vi "Fgen Arb Sequence.vi"() -> ()   [LabVIEW 2021]
doc: "This example shows how to use Arbitrary Sequence mode. It also shows how you can associate a name with each buffer you are generating."
uses:
  <instrlib>/niFgen/niFgen.llb/niFgen Output Mode.ctl
  <instrlib>/niFgen/niFgen.llb/niFgen_ctl Trigger SW - TrigName Values (Ring).ctl
  <instrlib>/niFgen/niFgen.llb/niFgen Disable Start Trigger.vi
  <instrlib>/niFgen/niFgen.llb/niFgen Configure Software Edge Start Trigger.vi
  <instrlib>/niFgen/niFgen.llb/niFgen Configure Digital Edge Start Trigger.vi
  <instrlib>/niFgen/niFgen.llb/niFgen Create Waveform (I16).vi
panel:
  in  "FGEN Resource Name":refnum<k15>
  in  "Re-Sequence":bool
  in  "Load & Re-Sequence":bool
  out "Resulting Sequence":string[](array[string])
  in  "Digital Filter":bool
  in  "Analog Filter":bool
  in  "DC Offset (V)":dbl(knob) scale=-0.5..0.5 scale format="%#.1f"
  in  "Gain":dbl(knob)=1.0 min=0.0 max=5.0 scale=0.0..5.0 scale format="%#.1f"
  in  "Send Software Trigger":bool
  in  "Sample Clock Source":string(combo)="OnboardClock"
  in  "Clock Mode":u32(ring)=1 items=["Hi Resolution Sampling", "Divide Down Sampling", "Automatic"]
  in  "Trigger Mode":u16(ring)=1 items=["Single", "Continuous", "Stepped", "Burst"]
  in  "Start Trigger Source":string(combo)="PFI0"
  in  "Start Trigger Type":u16(ring) items=["None", "Software Edge", "Digital Edge"]
  in  "Sample Rate":dbl=20000000.0 format="%.2p"
  in  "Sequence":T1(array[cluster])=[{"Waveform Name"=0, "# Loops"=1, "Marker"=-1}, {"Waveform Name"=1, "# Loops"=1, "Marker"=-1}, {"Waveform Name"=2, "# Loops"=3, "Marker"=-1}, {"Waveform Name"=3, "# Loops"=1, "Marker"=-1}] {"Waveform Name" items=["0: Big Ramp", "1: Small Sine", "2: Half Sized Square", "3: DC 0V"]}
  in  "Waveform Information Array":T2(array[cluster])=[{"Name"="Big Ramp", "Waveform"={"Waveform Type"=5, "Amplitude"=1.0, "# of points"=256}}, {"Name"="Small Sine", "Waveform"={"Waveform Type"=0, "Amplitude"=0.5, "# of points"=256}}, {"Name"="Half Sized Square", "Waveform"={"Waveform Type"=3, "Amplitude"=0.5, "# of points"=256}}, {"Name"="DC 0V", "Waveform"={"Waveform Type"=7, "Amplitude"=0.0, "# of points"=256}}] {"Waveform"."Amplitude" min=0.0 max=1.0 format="%.2f"; "Waveform"."Waveform Type" items=["Sine", "Cosine", "Triangle", "Square", "Sawtooth", "Increasing Ramp", "Decreasing Ramp", "DC Value"]}
  in  "Stop Button":bool
  # "Overview: Demonstrates how to configure an NI Arbitrary Waveform Generator to generate an arbitrary waveform with Arbitrary Sequence Mode. This example also demonstrates how to change the sequence without having to reload waveforms to onboard memory\nSoftware Requirements: NI-FGEN\nHardware Requirements: PXI-5411, PCI-5411, AT-5411, PXI-5412, PCI-5412, PXIe-5413, PXI-5421, PCI-5421, PXI-5422, PXIe-5423, PXI-5431, PCI-5431, PXIe-5433, PXI-5441, NI PXIe-5442, NI PXIe-5450, or NI PXIe-5451 \nInstructions:\n1. Select the FGEN Resource Name as configured in the Measurement & Automation Explorer.\n2. Specify the waveforms that will be generated in the Waveform Information Array.\n3. Specify the Sequence that you want to link and loop the waveforms specified in the Waveform Information Array.\n4. Specify the Gain and DC Offset that will be used.\n5. Specify the Sample Rate, Sample Clock Source, and  Clock Mode that will be used.\n6. Select the Start Trigger Type, Trigger Mode, and Start Trigger Source that will be used.\n7. Determine whether to enable the Analog Filter and/or the Digital Filter. \n8. Run the VI.\n9. Click Send Software Trigger to send a trigger if you have selected a relevant Start Trigger Type.\n10. You can change the Gain or DC Offset (V) values on-the-fly. You can also toggle the Analog Filter on-the-fly.\n11. Click Load & Re-Sequence to abort the generation and to load the waveforms from the Waveform Information Array and the Sequence to the device's onboard memory.\n12. Click Re-Sequence to abort the generation and to load the Sequence to the device's onboard memory.\n13. Click Stop to stop the VI."
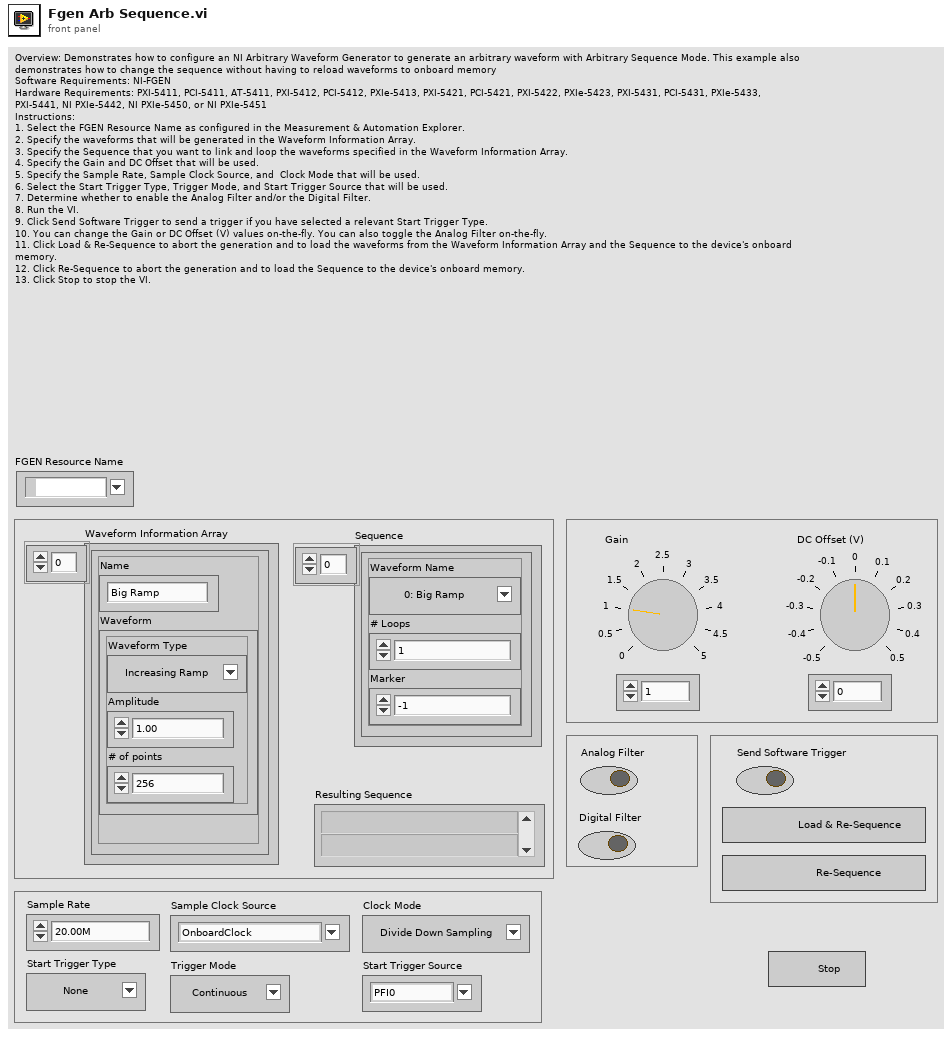
[diagram p1: front panel]
types:
  T1 = cluster{"Waveform Name":u16, "# Loops":i32, "Marker":i32}[]
  T2 = cluster{"Name":string, "Waveform":cluster{"Waveform Type":u16, "Amplitude":dbl, "# of points":u32}}[]
  T3 = typedef "niFgen Output Mode.ctl" = u32
  T4 = cluster{"Waveform Type":u16, "Amplitude":dbl, "# of points":u32}
  T5 = typedef "niFgen_ctl Trigger SW - TrigName Values (Ring).ctl" = i32
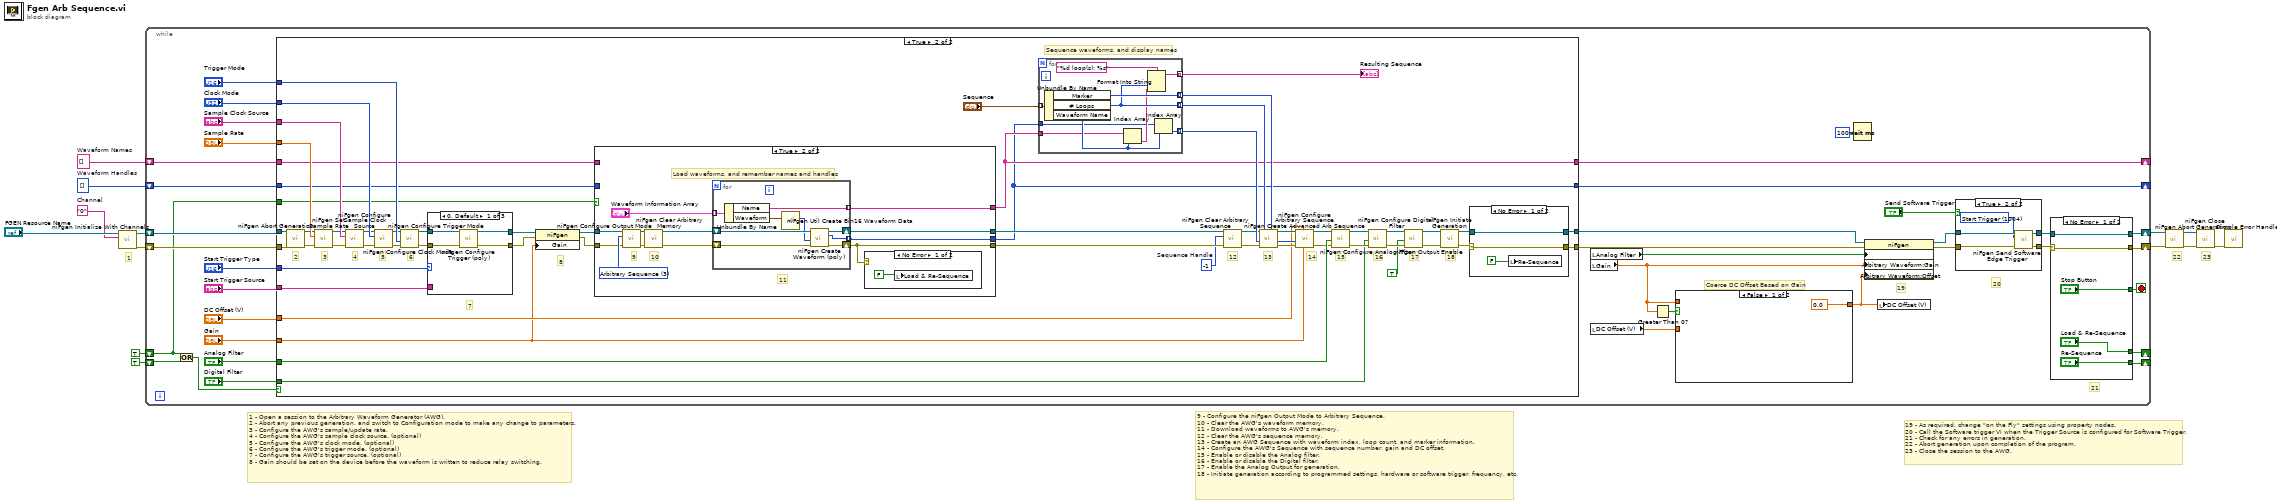
[diagram p0: block diagram]
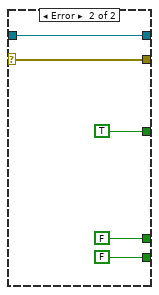
[diagram p2: hidden frame]
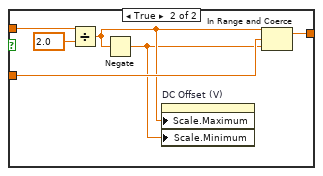
[diagram p3: hidden frame]
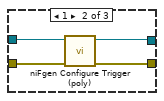
[diagram p9: hidden frame]
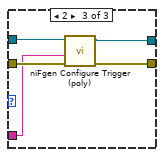
[diagram p10: hidden frame]
diagram:
  w1 = "0"  # Channel
  w9 = i32[] []  # Waveform Handles
  w10 = string[] []  # Waveform Names
  # "1"
  # "23"
  # "22"
  # "19 - As required, change \"on the Fly\" settings using property nodes.\n20 - Call the Software trigger VI when the Trigger Source is configured for Software Trigger.\n21 - Check for any errors in generation.\n22 - Abort generation upon completion of the program. \n23 - Close the session to the AWG."
  # "9 - Configure the niFgen Output Mode to Arbitrary Sequence.\n10 - Clear the AWG's waveform memory.\n11 - Download waveforms to AWG's memory.\n12 - Clear the AWG's sequence memory.\n13 - Create an AWG Sequence with waveform index, loop count, and marker information.\n14 - Configure the AWG's Sequence with sequence number, gain and DC offset.\n15 - Enable or disable the Analog filter.\n16 - Enable or disable the Digital filter.\n17 - Enable the Analog Output for generation.\n18 - Initiate generation according to programmed settings, hardware or software trigger, frequency, etc."
  # "1 - Open a session to the Arbitrary Waveform Generator (AWG).\n2 - Abort any previous generation, and switch to Configuration mode to make any change to parameters.\n3 - Configure the AWG's sample/update rate.\n4 - Configure the AWG's sample clock source. (optional)\n5 - Configure the AWG's clock mode. (optional)\n6 - Configure the AWG's trigger mode. (optional)\n7 - Configure the AWG's trigger source. (optional)\n8 - Gain should be set on the device before the waveform is written to reduce relay switching."
  n1 = call <instrlib>:"niFgen Initialize With Channels.vi"("Channel Name"=w1, "Resource Name"="FGEN Resource Name") -> ("error out"=w2:errorcluster, "Instrument Handle Out"=w3:refnum<k15>)  [unwired: 8 in]
  n2 = while {
    shift-left: TRUE ("Stop Button") -> [w49]
    shift-right: [w27] -> _
    shift-left: TRUE ("Stop Button") -> [w42]
    shift-right: [w28] -> _
    shift-left: w9 -> [w41]
    shift-right: [w38] -> _
    shift-right: [w15] -> w11
    shift-left: w2 -> [w43]
    shift-right: [w39] -> _
    shift-left: w10 -> [w40]
    shift-right: [w16] -> w8
    shift-left: w3 -> [w44]
    stop <- w26 stop-if-true
    # "20"
    # "19"
    # "Coerce DC Offset Based on Gain"
    # "21"
    n3 = Or(x=w42, y=w49) -> (x .or. y?=w50:bool)
    n4 = case shown="True" w50 {
      tunnel: w43 -> [w75 w117]
      tunnel: [w78 w90] -> w37
      tunnel: [w75 w91] -> w36
      tunnel: w44 -> [w78 w116]
      tunnel: "Analog Filter" -> [_ w120]
      tunnel: "Gain" -> [_ w79]
      tunnel: "Sample Rate" -> [_ w106]
      tunnel: "DC Offset (V)" -> [_ w119]
      tunnel: "Start Trigger Type" -> [_ w110]
      tunnel: "Trigger Mode" -> [_ w118]
      tunnel: "Clock Mode" -> [_ w112]
      tunnel: "Digital Filter" -> [_ w115]
      tunnel: "Sample Clock Source" -> [_ w114]
      tunnel: "Start Trigger Source" -> [_ w109]
      tunnel: w42 -> [_ w97]
      tunnel: w41 -> [w76 w95]
      tunnel: w40 -> [w77 w96]
      tunnel: [w77 w94] -> w39
      tunnel: [w76 w85] -> w38
      frame False {
      }
      frame True {
        w87 = -1  # Sequence Handle
        # "8"
        # "Sequence waveforms, and display names"
        # "18"
        # "17"
        # "16"
        # "15"
        # "14"
        # "13"
        # "12"
        # "6"
        # "5"
        # "4"
        # "3"
        # "2"
        # "7"
        n5 = call <instrlib>:"niFgen Abort Generation.vi"("error in (no error)"=w117, "Instrument Handle"=w116) -> ("error out"=w104:errorcluster, "Instrument Handle Out"=w105:refnum<k15>)  [unwired: 8 in]
        n6 = call <instrlib>:"niFgen Set Sample Rate.vi"("error in (no error)"=w104, "Sample Rate (Samp/s)"=w106, "Instrument Handle"=w105) -> ("error out"=w103:errorcluster, "Instrument Handle Out"=w100:refnum<k15>)  [unwired: 7 in]
        n7 = call <instrlib>:"niFgen Configure Sample Clock Source.vi"("error in (no error)"=w103, "Source (Onboard Clock)"=w114, "Instrument Handle"=w100) -> ("error out"=w102:errorcluster, "Instrument Handle Out"=w101:refnum<k15>)  [unwired: 7 in]
        n8 = call <instrlib>:"niFgen Configure Clock Mode.vi"("error in (no error)"=w102, "Clock Mode (default: 1=divide down)"=w112, "Instrument Handle"=w101) -> ("error out"=w111:errorcluster, "Instrument Handle Out"=w113:refnum<k15>)  [unwired: 7 in]
        n9 = call <instrlib>:"niFgen Configure Trigger Mode.vi"("error in (no error)"=w111, "Trigger Mode (default: 1=continuous)"=w118, "Instrument Handle"=w113) -> ("error out"=w130:errorcluster, "Instrument Handle Out"=w81:refnum<k15>)  [unwired: 7 in]
        n10 = case shown="0, Default" w110 {
          tunnel: w130 -> [w170 w174 w179]
          tunnel: [w169 w173 w178] -> w82
          tunnel: w109 -> [_ _ w177]
          tunnel: w81 -> [w168 w172 w176]
          tunnel: [w167 w171 w175] -> w80
          frame 0, Default {
            n11 = call-poly <instrlib>:"niFgen Configure Trigger (poly).vi"("error in (no error)"=w170, "Instrument Handle"=w168) -> ("error out"=w169:errorcluster, "Instrument Handle Out"=w167:refnum<k15>)  [unwired: 8 in]
          }
          frame 1 {
            n12 = call-poly <instrlib>:"niFgen Configure Trigger (poly).vi"("error in (no error)"=w174, "Instrument Handle"=w172) -> ("error out"=w173:errorcluster, "Instrument Handle Out"=w171:refnum<k15>)  [unwired: 8 in]
          }
          frame 2 {
            n13 = call-poly <instrlib>:"niFgen Configure Trigger (poly).vi"("error in (no error)"=w179, "Source"=w177, "Instrument Handle"=w176) -> ("error out"=w178:errorcluster, "Instrument Handle Out"=w175:refnum<k15>)  [unwired: 7 in]
          }
        }
        n14 = property class="niFgen"(reference=w80, error in=w82, "Gain"=w79) -> (reference out=w84:refnum<k15>, error out=w83:errorcluster)
        n15 = case shown="True" w97 {
          tunnel: w84 -> [w144 w153]
          tunnel: w83 -> [w143 w152]
          tunnel: [w143 w149] -> w99
          tunnel: [w144 w147] -> w98
          tunnel: [w141 w151] -> w94
          tunnel: [w142 w148] -> w85
          tunnel: w96 -> [w141 _]
          tunnel: w95 -> [w142 _]
          frame False {
          }
          frame True {
            w154 = T3 3 items=["Standard Function", "Frequency List", "Arbitrary Waveform", "Arbitrary Sequence", "Script"] ("Output Mode")
            # "11"
            # "10"
            # "9"
            # "Load waveforms, and remember names and handles"
            n16 = call <instrlib>:"niFgen Configure Output Mode.vi"("error in (no error)"=w152, "Output Mode (default: 0=Standard Function)"=w154, "Instrument Handle"=w153) -> ("error out"=w155:errorcluster, "Instrument Handle Out"=w156:refnum<k15>)  [unwired: 6 in]
            n17 = call <instrlib>:"niFgen Clear Arbitrary Memory.vi"("error in (no error)"=w155, "Instrument Handle"=w156) -> ("error out"=w146:errorcluster, "Instrument Handle Out"=w145:refnum<k15>)  [unwired: 8 in]
            n18 = for {
              shift-right: [w165] -> w149
              shift-left: w146 -> [w163]
              tunnel: [w158] -> w148 mode=indexing
              shift-right: [w166] -> w147
              shift-left: w145 -> [w164]
              tunnel: [w159] -> w151 mode=indexing
              tunnel: "Waveform Information Array" -> [w160] mode=indexing
              n19 = Unbundle By Name(w160) -> ("Name"=w159:string, "Waveform"=w162:T4)
              n20 = call <instrlib>:"niFgen Util Create Bin16 Waveform Data.vi"("Waveform"=w162) -> ("Waveform Data"=w161:i16[])  [unwired: 10 in]
              n21 = call-poly <instrlib>:"niFgen Create Waveform (poly).vi"("error in (no error)"=w163, "Waveform Data Array"=w161, "Instrument Handle"=w164) -> ("error out"=w165:errorcluster, "Waveform Handle"=w158:i32, "Instrument Handle Out"=w166:refnum<k15>)  [unwired: 6 in]
            }
            n22 = case shown="No Error" w149 {
              frame No Error {
                n23 = local write "Load & Re-Sequence"(FALSE ("Load?")) -> ()
              }
              frame Error {
              }
            }
          }
        }
        n24 = for {
          tunnel: "Sequence" -> [w189] mode=indexing
          tunnel: [w187] -> w132 mode=indexing
          tunnel: [w188] -> w124 mode=indexing
          tunnel: [w185] -> w123 mode=indexing
          tunnel: [w184] -> w88 mode=indexing
          tunnel: w94 -> [w182]
          tunnel: w85 -> [w180]
          n25 = Unbundle By Name(w189) -> ("Marker"=w188:i32, "# Loops"=w185:i32, "Waveform Name"=w183:u16)
          n26 = Index Array(array=w182, index=w183) -> (element=w181:string)
          n27 = Format Into String(format string="%d loop(s): %s", w185, w181) -> (resulting string=w184:string)  [unwired: 2 in, 1 out]
          n28 = Index Array(array=w180, index=w183) -> (element=w187:i32)
        }
        "Resulting Sequence" <- w88
        n29 = call <instrlib>:"niFgen Clear Arbitrary Sequence.vi"("error in (no error)"=w99, "Sequence Handle"=w87, "Instrument Handle"=w98) -> ("error out"=w129:errorcluster, "Instrument Handle Out"=w131:refnum<k15>)  [unwired: 7 in]
        n30 = call <instrlib>:"niFgen Create Advanced Arb Sequence.vi"("Marker Location Array"=w124, "Loop Counts Array"=w123, "error in (no error)"=w129, "Waveform Handles Array"=w132, "Instrument Handle"=w131) -> ("error out"=w135:errorcluster, "Sequence Handle"=w134:i32, "Instrument Handle Out"=w133:refnum<k15>)  [unwired: 3 in, 1 out]
        n31 = call <instrlib>:"niFgen Configure Arbitrary Sequence.vi"("Gain"=w79, "Offset"=w119, "error in (no error)"=w135, "Sequence Handle"=w134, "Instrument Handle"=w133) -> ("error out"=w107:errorcluster, "Instrument Handle Out"=w108:refnum<k15>)  [unwired: 5 in]
        n32 = call <instrlib>:"niFgen Configure Analog Filter.vi"("error in (no error)"=w107, "Analog Filter Enable (default: True)"=w120, "Instrument Handle"=w108) -> ("error out"=w128:errorcluster, "Instrument Handle Out"=w126:refnum<k15>)  [unwired: 7 in]
        n33 = call <instrlib>:"niFgen Configure Digital Filter.vi"("error in (no error)"=w128, "Digital Filter Enable (default: True)"=w115, "Instrument Handle"=w126) -> ("error out"=w127:errorcluster, "Instrument Handle Out"=w125:refnum<k15>)  [unwired: 7 in]
        n34 = call <instrlib>:"niFgen Output Enable.vi"("error in (no error)"=w127, "Output Enable (default: True)"=TRUE ("output enable"), "Instrument Handle"=w125) -> ("error out"=w121:errorcluster, "Instrument Handle Out"=w122:refnum<k15>)  [unwired: 7 in]
        n35 = call <instrlib>:"niFgen Initiate Generation.vi"("error in (no error)"=w121, "Instrument Handle"=w122) -> ("error out"=w92:errorcluster, "Instrument Handle Out"=w89:refnum<k15>)  [unwired: 8 in]
        n36 = case shown="No Error" w92 {
          selector: w92 -> [w138 w139]
          tunnel: [w138 w139] -> w91
          tunnel: [w137 w140] -> w90
          tunnel: w89 -> [w137 w140]
          frame No Error {
            n37 = local write "Re-Sequence"(FALSE ("Sequence?")) -> ()
          }
          frame Error {
          }
        }
      }
    }
    n38 = local read "Analog Filter"() -> (w19:bool)
    n39 = local read "Gain"() -> (w22:dbl)
    n40 = local read "DC Offset (V)"() -> (w23:dbl)
    n41 = Greater Than 0?(x=w22) -> (x > 0?=w46:bool)
    n42 = case shown="False" w46 {
      tunnel: w22 -> [_ w67]
      tunnel: w23 -> [_ w66]
      tunnel: [0.0 ("DC Offset") w65] -> w18
      frame False {
      }
      frame True {
        n43 = Divide(x=w67, y=2.0) -> (x/y=w64:dbl)
        n44 = Negate(x=w64) -> (-x=w63:dbl)
        n45 = property on="DC Offset (V)" class="Knob (strict)"("Scale.Maximum"=w64, "Scale.Minimum"=w63) -> ()  [unwired: 2 in, 2 out]
        n46 = In Range and Coerce(upper limit=w64, x=w66, lower limit=w63) -> (coerced(x)=w65:dbl)  [unwired: 1 out]
      }
    }
    n47 = Wait (ms)(milliseconds to wait=u32 100 ("delay")) -> ()  [unwired: 1 out]
    n48 = property class="niFgen"(reference=w37, error in=w36, "Output:Filters:Analog Filter Enabled"=w19, "Arbitrary Waveform:Gain"=w22, "Arbitrary Waveform:Offset"=w18) -> (reference out=w48:refnum<k15>, error out=w47:errorcluster)
    n49 = local write "DC Offset (V)"(w18) -> ()
    n50 = case shown="True" "Send Software Trigger" {
      tunnel: w48 -> [w69 w74]
      tunnel: [w69 w73] -> w17
      tunnel: w47 -> [w68 w70]
      tunnel: [w68 w72] -> w14
      frame False {
      }
      frame True {
        w71 = T5 1004 items=["Start Trigger"=1004, "Script Trigger"=104] ("Trigger (Start Trigger)")
        n51 = call <instrlib>:"niFgen Send Software Edge Trigger.vi"("error in (no error)"=w70, "Trigger (Start Trigger)"=w71, "Instrument Handle"=w74) -> ("error out"=w72:errorcluster, "Instrument Handle Out"=w73:refnum<k15>)  [unwired: 7 in]
      }
    }
    n52 = case shown="No Error" w14 {
      selector: w14 -> [w54 w60]
      tunnel: [w55 w59] -> w16
      tunnel: w17 -> [w55 w59]
      tunnel: [w54 w60] -> w15
      tunnel: ["Stop Button" TRUE ("Stop Button")] -> w26
      tunnel: ["Load & Re-Sequence" FALSE ("Stop Button")] -> w28
      tunnel: ["Re-Sequence" FALSE ("Stop Button")] -> w27
      frame No Error {
      }
      frame Error {
      }
    }
  }
  n53 = call <instrlib>:"niFgen Abort Generation.vi"("error in (no error)"=w11, "Instrument Handle"=w8) -> ("error out"=w12:errorcluster, "Instrument Handle Out"=w13:refnum<k15>)  [unwired: 8 in]
  n54 = call <instrlib>:"niFgen Close.vi"("error in (no error)"=w12, "Instrument Handle"=w13) -> ("error out"=w7:errorcluster)  [unwired: 9 in]
  n55 = call <vilib>:"Simple Error Handler.vi"("error in (no error)"=w7) -> ()  [unwired: 4 in, 5 out]
